vi "Create PUBCOMP Packet.vi"(5 "PUBCOMP in":refnum<class "PUBCOMP.lvclass">, 8 "error in (no error)":errorcluster, 9 "Packet ID":u16 format="%04x") -> (0 "error out":errorcluster, 2 "Bytes Stream":u8[](array[numeric]) format="%08b", 3 "PUBCOMP out":refnum<class "PUBCOMP.lvclass">)   [LabVIEW 2013, in "MQTT_Control_Packets.lvlib" / "PUBCOMP.lvclass"]
uses:
  PUBCOMP.lvclass
  ControlPacket/ControlPacket.lvclass/ControlPacket.ctl
  ControlPacket/ControlPacket.lvclass
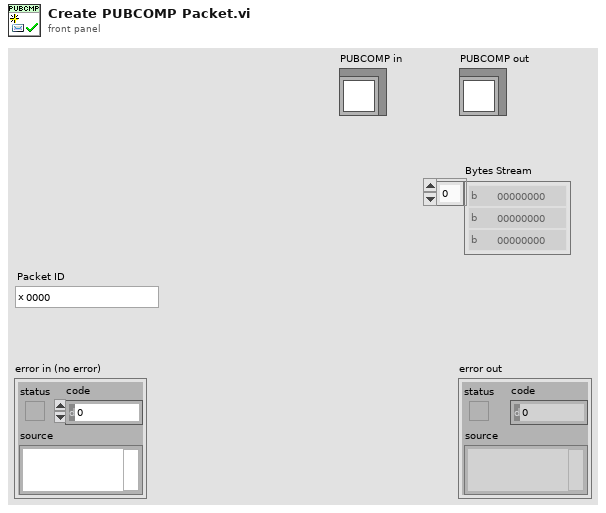
[diagram p1: front panel]
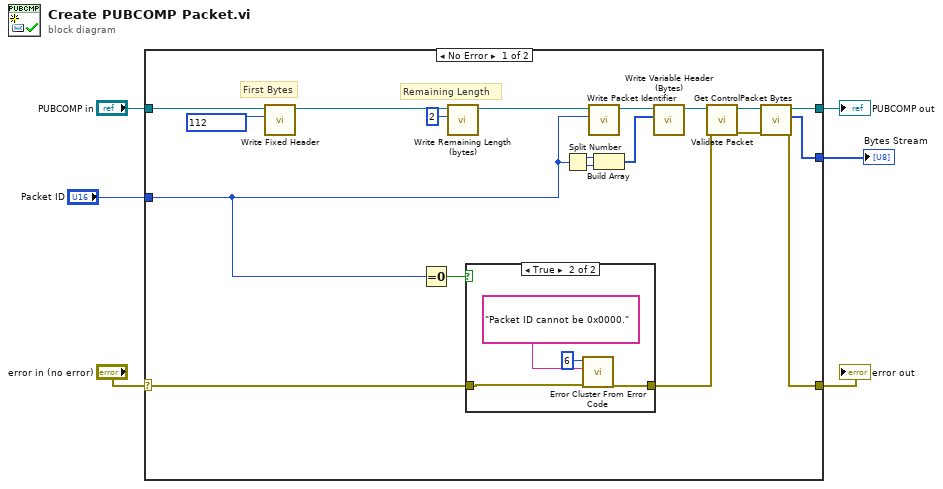
[diagram p0: block diagram]
diagram:
  n1 = case shown="No Error" "error in (no error)" {
    selector: "error in (no error)" -> [w14 w32]
    tunnel: [w8 w32] -> w3
    tunnel: [w10 w31] -> w2
    tunnel: "PUBCOMP in" -> [w25 w31]
    tunnel: "Packet ID" -> [w16 _]
    tunnel: [w7 _] -> w1
    frame No Error {
      # "Remaining Length"
      # "First Bytes"
      n2 = call "Write Fixed Header.vi"("Fixed Header"=u8 112, "ControlPacket in"=w25) -> ("ControlPacket out"=w24:refnum<class "PUBCOMP.lvclass">)  [unwired: 9 in]
      n3 = Equal To 0?(x=w16) -> (x = 0?=w15:bool)
      n4 = call "Write Remaining Length (bytes).vi"("Remaining Length (bytes)"=u32 2, "ControlPacket in"=w24) -> ("ControlPacket out"=w20:refnum<class "PUBCOMP.lvclass">)  [unwired: 9 in]
      n5 = case shown="True" w15 {
        tunnel: w14 -> [w26 w29]
        tunnel: [w26 w30] -> w11
        frame False {
        }
        frame True {
          n6 = call <vilib>:"Error Cluster From Error Code.vi"("error in (no error)"=w29, "error message (\"\")"="Packet ID cannot be 0x0000.", "error code (0)"=6) -> ("error out"=w30:errorcluster)  [unwired: 6 in]
        }
      }
      n7 = Split Number(x=w16) -> (hi(x)=w23:u8, lo(x)=w22:u8)
      n8 = call "Write Packet Identifier.vi"("Packet Identifier"=w16, "ControlPacket in"=w20) -> ("ControlPacket out"=w19:refnum<class "PUBCOMP.lvclass">)  [unwired: 9 in]
      n9 = Build Array(w23, w22) -> (w21:u8[])
      n10 = call "Write Variable Header (Bytes).vi"("Variable Header (Bytes)"=w21, "ControlPacket in"=w19) -> ("ControlPacket out"=w13:refnum<class "PUBCOMP.lvclass">)  [unwired: 9 in]
      n11 = call "Validate Packet.vi"("error in (no error)"=w11, "ControlPacket in"=w13) -> ("error out"=w9:errorcluster, "ControlPacket out"=w12:refnum<class "PUBCOMP.lvclass">)  [unwired: 8 in]
      n12 = call "Get ControlPacket Bytes.vi"("error in (no error)"=w9, "ControlPacket"=w12) -> ("error out"=w8:errorcluster, "Bytes Stream"=w7:u8[], "ControlPacket dup"=w10:refnum<class "PUBCOMP.lvclass">)  [unwired: 6 in, 1 out]
    }
    frame Error {
    }
  }
  "error out" <- w3
  "PUBCOMP out" <- w2
  "Bytes Stream" <- w1
